vi "LearningVI_3_wOutput.vi"() -> ()   [LabVIEW 2013]
panel:
  in  "Output 2V \non AO-0":bool
  in  "STOP":bool
  in  "Save Waveform":bool
  out "DC t-Avg":dbl[](array[numeric])
  out "Peak2Peak V":dbl[](array[numeric])
  out "Waveform Chart":dynamicdata(graph)
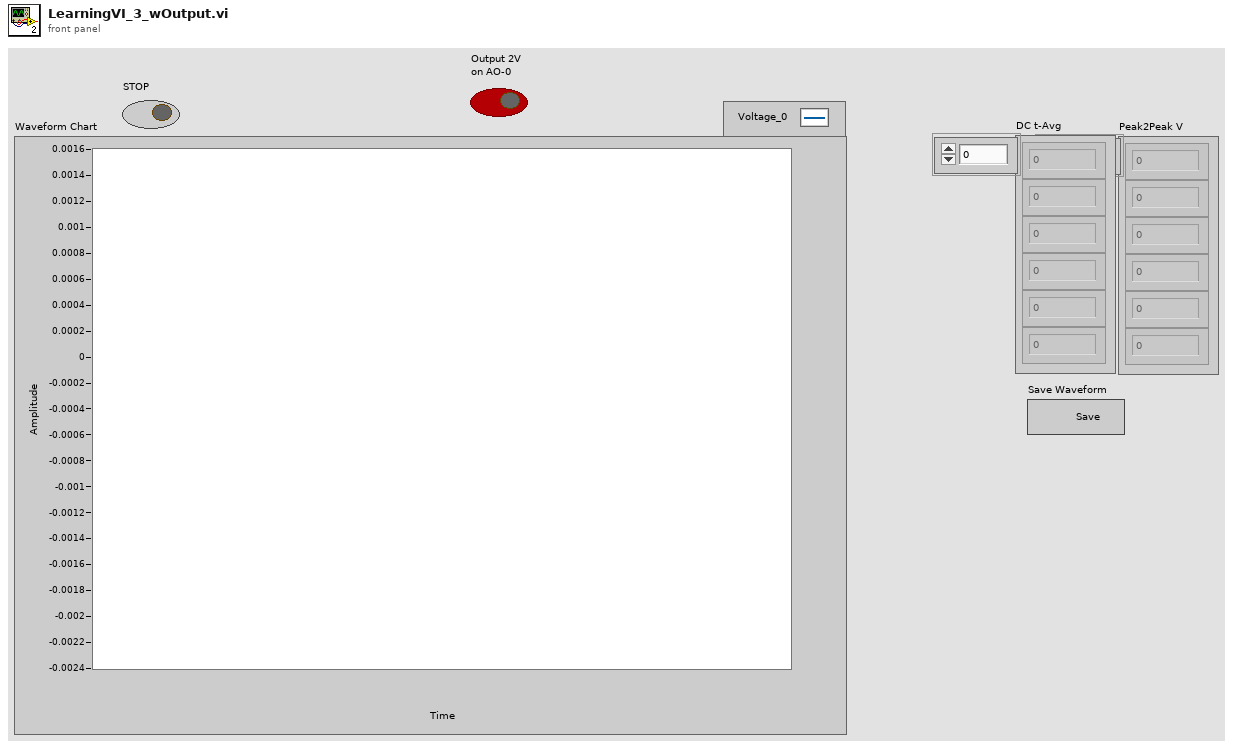
[diagram p1: front panel]
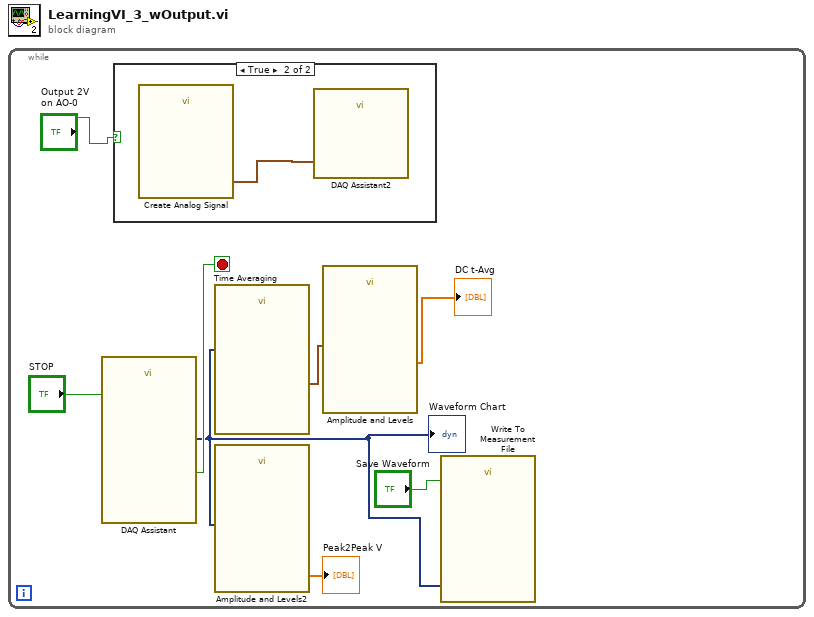
[diagram p0: block diagram]
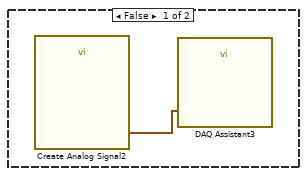
[diagram p2: hidden frame]
diagram:
  n1 = while {
    stop <- w8 stop-if-true
    n2 = call "DAQ Assistant"("stop (F)"="STOP") -> ("data"=w4:dynamicdata, "stopped"=w8:bool)  [unwired: 15 in, 2 out]
    "Waveform Chart" <- w4
    n3 = case shown="True" "Output 2V \non AO-0" {
      frame False {
        n4 = call "Create Analog Signal2"() -> ("DC signal"=w9:waveform(dbl))  [unwired: 18 in, 1 out]
        n5 = call "DAQ Assistant3"("data"=w9) -> ()  [unwired: 17 in, 2 out]
      }
      frame True {
        n6 = call "Create Analog Signal"() -> ("DC signal"=w10:waveform(dbl))  [unwired: 18 in, 1 out]
        n7 = call "DAQ Assistant2"("data"=w10) -> ()  [unwired: 17 in, 2 out]
      }
    }
    n8 = call "Time Averaging"("input signals"=w4) -> ("time avg. signal"=w7:waveform(dbl)[])  [unwired: 15 in, 3 out]
    n9 = call "Amplitude and Levels2"("input signals"=w4) -> ("peak-peak"=→"Peak2Peak V":dbl[])  [unwired: 15 in, 3 out]
    n10 = call "Amplitude and Levels"("input signals"=w7) -> ("dc"=→"DC t-Avg":dbl[])  [unwired: 15 in, 3 out]
    n11 = call "Write To Measurement File"("Signals"=w4, "Enable"="Save Waveform") -> ()  [unwired: 15 in, 3 out]
  }
